vi "Wavefrom Subsets from Cursors Single.vi"(8 "Error In":errorcluster, 9 "Waveforms In":waveform(dbl)[](array[waveform]), 11 "Waveform Graph":refnum<vi>) -> (0 "Error Out":errorcluster, 1 "Waveform Subsets":waveform(dbl)[](array[waveform]))   [LabVIEW 2019]
uses:
  <vilib>/Waveform/WDTOps.llb/WDT Waveform Duration DBL.vi
  <vilib>/Waveform/WDTOps.llb/WDT Get Waveform Subset DBL.vi
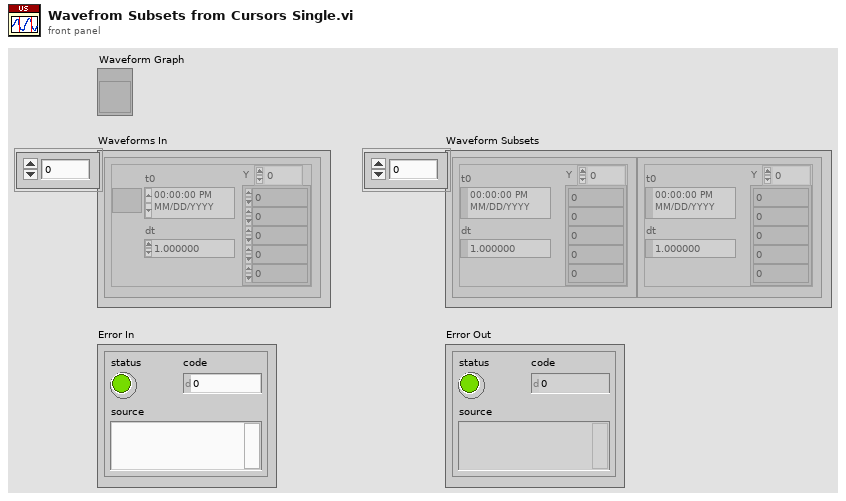
[diagram p1: front panel]
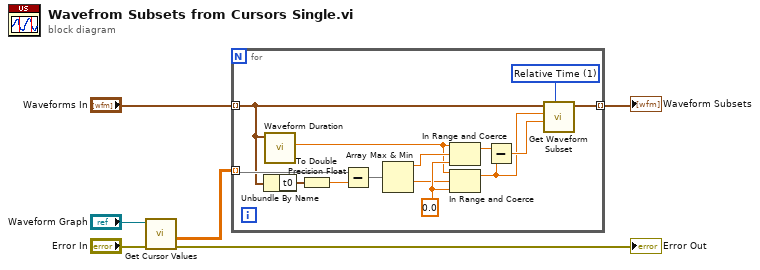
[diagram p0: block diagram]
diagram:
  n1 = call "Get Cursor Values.vi"("error in (no error)"="Error In", "Waveform Graph Ref"="Waveform Graph") -> ("error out"=→"Error Out":errorcluster, "Cursor values"=w6:dbl[][])  [unwired: 7 in]
  n2 = for {
    tunnel: w6 -> [w13] mode=indexing
    tunnel: "Waveforms In" -> [w7] mode=indexing
    tunnel: [w11] -> w2 mode=indexing
    w16 = 0.0 ("lower limit")
    w12 = u16 1 items=["Samples", "Relative Time"] ("start/duration format")
    n3 = Unbundle By Name(w7) -> ("t0"=w10:timestamp)
    n4 = call-poly <vilib>:"Waveform Duration.vi"("waveform in"=w7) -> ("duration"=w8:dbl)  [unwired: 8 in, 2 out]
    n5 = To Double Precision Float(number=w10) -> (double precision float=w9:dbl)
    n6 = Subtract(x=w13, y=w9) -> (x-y=w14:dbl[])
    n7 = Array Max & Min(array=w14) -> (max value=w17:dbl, min value=w15:dbl)  [unwired: 2 out]
    n8 = In Range and Coerce(upper limit=w8, x=w17, lower limit=w16) -> (coerced(x)=w18:dbl)  [unwired: 1 out]
    n9 = In Range and Coerce(upper limit=w8, x=w15, lower limit=w16) -> (coerced(x)=w19:dbl)  [unwired: 1 out]
    n10 = Subtract(x=w18, y=w19) -> (x-y=w20:dbl)
    n11 = call-poly <vilib>:"Get Waveform Subset.vi"("start/duration format"=w12, "duration"=w20, "start samples/time"=w19, "waveform in"=w7) -> ("waveform out"=w11:waveform(dbl))  [unwired: 2 in, 3 out]
  }
  "Waveform Subsets" <- w2
